vi "CreateInterface.vi"(6 "InterfaceName":string, 7 "Application":refnum<vi>, 8 "error in":errorcluster, 9 "Interface Folder":path, 10 "Parent Interfaces(ClassRef/Path)":variant[](array[variant]), 11 "New Interface Owner":refnum<vi>) -> (0 "error out":errorcluster, 1 "Interface":refnum<vi>, 2 "InterfaceName(Qualified Name)":string, 3 "InterfaceName(Non Qualified)":string, 4 "InterfacePath":path)   [LabVIEW 2020, in "InterfaceLibrary.lvlib"]
uses:
  <resource>/Framework/Providers/Open_GDS/ClassProviders/Common/InterfaceLibrary/InterfaceLibrary.lvlib
  <vilib>/numeric/Random Number (Range) U64.vi
  <vilib>/numeric/sub_Random U32.vi
  <resource>/Framework/Providers/_ClassSupport/Class Provider Support.lvlib
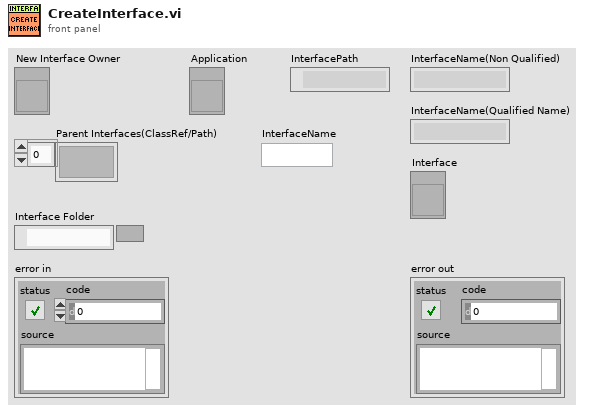
[diagram p1: front panel]
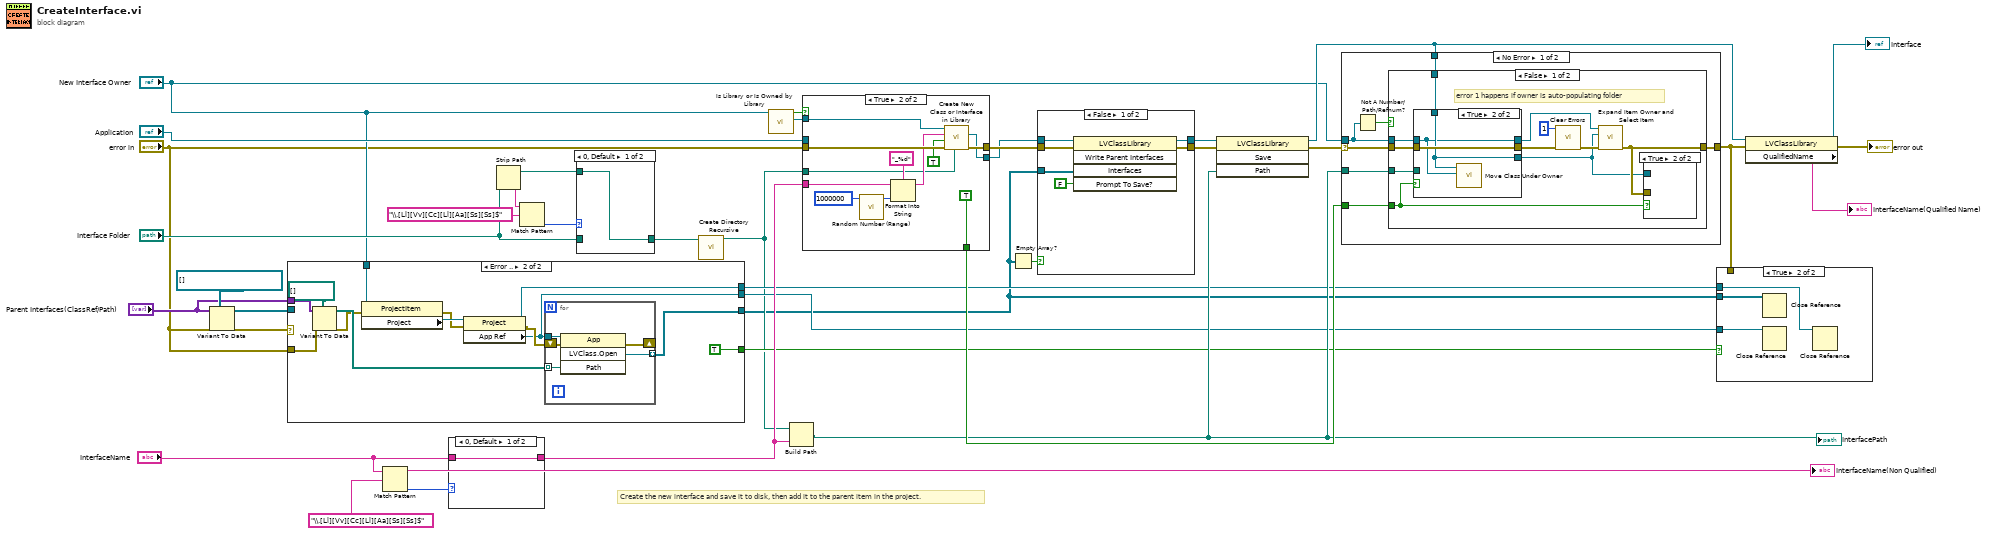
[diagram p0: block diagram]
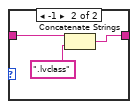
[diagram p4: hidden frame]
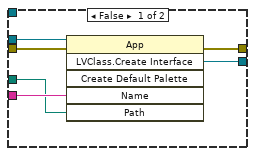
[diagram p6: hidden frame]
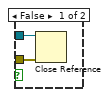
[diagram p7: hidden frame]
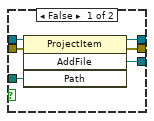
[diagram p8: hidden frame]
diagram:
  # "Create the new interface and save it to disk, then add it to the parent item in the project."
  n1 = Variant To Data(error in="error in", type=refnum<vi>[] [] ("Interface"), Variant="Parent Interfaces(ClassRef/Path)") -> (data=w11:refnum<vi>[], error out=w12:errorcluster)
  n2 = case shown="Error .." w12 {
    tunnel: [w39 w43] -> w1
    tunnel: w11 -> [w39 _]
    tunnel: "Parent Interfaces(ClassRef/Path)" -> [_ w51]
    tunnel: "New Interface Owner" -> [_ w50]
    tunnel: "error in" -> [_ w44]
    tunnel: [_ w42] -> w7
    tunnel: [_ w41] -> w6
    tunnel: [_ TRUE] -> w4
    frame No Error {
    }
    frame Error {
      n3 = Variant To Data(error in=w44, type=path[] [] ("Interface"), Variant=w51) -> (data=w48:path[], error out=w45:errorcluster)
      n4 = property class="ProjectItem"(reference=w50, error in=w45) -> (error out=w46:errorcluster, "Project"=w49:refnum<vi>)  [unwired: 1 out]
      n5 = property class="Project"(reference=w49, error in=w46) -> (reference out=w41:refnum<vi>, error out=w47:errorcluster, "App Ref"=w42:refnum<vi>)
      n6 = for {
        tunnel: w42 -> [w57]
        tunnel: w48 -> [w56] mode=indexing
        tunnel: [w54] -> w43 mode=indexing
        shift-right: [w53] -> _
        shift-left: w47 -> [w55]
        n7 = invoke class="App" method="LVClass.Open"(reference=w57, error in=w55, "Path"=w56) -> (error out=w53:errorcluster, "LVClass.Open"=w54:refnum<vi>)  [unwired: 1 in, 2 out]
      }
    }
  }
  n8 = Match Pattern(string="InterfaceName", regular expression="\\.[Ll][Vv][Cc][Ll][Aa][Ss][Ss]$") -> (before substring=→"InterfaceName(Non Qualified)":string, offset past match=w22:i32)  [unwired: 1 in, 2 out]
  n9 = case shown="0, Default" w22 {
    tunnel: "InterfaceName" -> [w58 w61]
    tunnel: [w58 w59] -> w20
    frame 0, Default {
    }
    frame -1 {
      n10 = Concatenate Strings(w61, ".lvclass" ("string")) -> (w59:string)
    }
  }
  n11 = Strip Path(path="Interface Folder") -> (stripped path=w24:path, name=w28:string)
  n12 = Match Pattern(string=w28, regular expression="\\.[Ll][Vv][Cc][Ll][Aa][Ss][Ss]$") -> (offset past match=w26:i32)  [unwired: 1 in, 3 out]
  n13 = case shown="0, Default" w26 {
    tunnel: "Interface Folder" -> [_ w63]
    tunnel: [w62 w63] -> w3
    tunnel: w24 -> [w62 _]
    frame 0, Default {
    }
    frame -1 {
    }
  }
  n14 = call <vilib>:"Create Directory Recursive.vi"("directory"=w3) -> ("directory copy"=w2:path)  [unwired: 4 in, 2 out]
  n15 = call <resource>:"Is Library or Is Owned by Library.vi"("ProjectItem"="New Interface Owner") -> ("Owning Library (or self)"=w33:refnum<vi>, "Is Library or Owned by Library?"=w32:bool)  [unwired: 9 in]
  n16 = Build Path(base path=w2, name or relative path=w20) -> (appended path=w14:path)
  "InterfacePath" <- w14
  n17 = case shown="True" w32 {
    tunnel: "error in" -> [w69 w81]
    tunnel: [w68 w80] -> w36
    tunnel: "Application" -> [w67 _]
    tunnel: w20 -> [w66 w75]
    tunnel: [w65 w78] -> w30
    tunnel: w33 -> [_ w79]
    tunnel: [_ TRUE] -> w29
    tunnel: w2 -> [w64 w70]
    frame False {
      n18 = invoke class="App" method="LVClass.Create Interface"(reference=w67, error in=w69, "Name"=w66, "Path"=w64) -> (error out=w68:errorcluster, "LVClass.Create Interface"=w65:refnum<vi>)  [unwired: 2 in, 4 out]
    }
    frame True {
      n19 = call-poly <vilib>:"Random Number (Range).vi"("upper bound (100)"=u64 1000000) -> ("number"=w72:u64)  [unwired: 10 in]
      n20 = Format Into String(format string="_%d", initial string=w75, w72) -> (resulting string=w74:string)  [unwired: 1 in, 1 out]
      n21 = call <vilib>:"Create New Class or Interface in Library.vi"("directory (empty)"=w70, "error in"=w81, "create interface"=TRUE, "new class file name"=w74, "library reference in"=w79) -> ("error out"=w80:errorcluster, "class reference"=w78:refnum<vi>)  [unwired: 4 in, 1 out]
    }
  }
  n22 = Empty Array?(array=w1) -> (empty?=w34:bool)
  n23 = case shown="False" w34 {
    tunnel: w36 -> [w87 w89]
    tunnel: [w86 w89] -> w37
    tunnel: w30 -> [w85 w88]
    tunnel: [w84 w88] -> w35
    tunnel: w1 -> [w82 _]
    frame False {
      n24 = invoke class="LVClassLibrary" method="Write Parent Interfaces"(reference=w85, error in=w87, "Interfaces"=w82, "Prompt To Save?"=FALSE) -> (reference out=w84:refnum<vi>, error out=w86:errorcluster)  [unwired: 1 in, 3 out]
    }
    frame True {
    }
  }
  n25 = invoke class="LVClassLibrary" method="Save"(reference=w35, error in=w37, "Path"=w14) -> (reference out=w17:refnum<vi>, error out=w38:errorcluster)  [unwired: 1 in, 2 out]
  n26 = case shown="No Error" w38 {
    selector: w38 -> [w96 w120]
    tunnel: "New Interface Owner" -> [w93 _]
    tunnel: w14 -> [w94 _]
    tunnel: [w95 w120] -> w5
    tunnel: w29 -> [w91 _]
    tunnel: w17 -> [w90 _]
    frame No Error {
      n27 = Not A Number/Path/Refnum?(number/path/refnum=w93) -> (NaN/Path/Refnum?=w92:bool)
      n28 = case shown="False" w92 {
        tunnel: w96 -> [w107 w119]
        tunnel: w94 -> [w102 _]
        tunnel: [w105 w119] -> w95
        tunnel: w93 -> [w99 _]
        tunnel: w91 -> [w97 _]
        tunnel: w90 -> [w98 _]
        frame False {
          # "error 1 happens if owner is auto-populating folder"
          n29 = case shown="True" w97 {
            tunnel: w107 -> [w115 w118]
            tunnel: [w114 w118] -> w106
            tunnel: [w113 w117] -> w103
            tunnel: w102 -> [w112 _]
            tunnel: [w111 w116] -> w101
            tunnel: w99 -> [w110 w116]
            tunnel: w98 -> [_ w117]
            frame False {
              n30 = invoke class="ProjectItem" method="AddFile"(reference=w110, error in=w115, "Path"=w112) -> (reference out=w111:refnum<vi>, error out=w114:errorcluster, "AddFile"=w113:refnum<vi>)  [unwired: 1 in, 1 out]
            }
            frame True {
              n31 = call <resource>:"Move Class Under Owner.vi"("Owner of New Class"=w116, "New Class"=w117) -> ()  [unwired: 9 in, 1 out]
            }
          }
          n32 = call <vilib>:"Clear Errors.vi"("error in (no error)"=w106, "specific error code to clear (0: all)"=1) -> ("error out"=w104:errorcluster)  [unwired: 4 in, 1 out]
          n33 = call <resource>:"Expand Item Owner and Select Item.vi"("error in"=w104, "New Item"=w103, "New Item Owner"=w101) -> ("error out"=w105:errorcluster)  [unwired: 8 in]
          n34 = case shown="True" w97 {
            tunnel: w105 -> [w109 _]
            tunnel: w103 -> [w108 _]
            frame False {
              n35 = Close Reference(reference=w108, error in (no error)=w109) -> ()  [unwired: 1 out]
            }
            frame True {
            }
          }
        }
        frame True {
        }
      }
    }
    frame Error {
    }
  }
  n36 = case shown="True" w4 {
    tunnel: w7 -> [_ w123]
    tunnel: w6 -> [_ w122]
    tunnel: w5 -> [_ _]
    tunnel: w1 -> [_ w121]
    frame False {
    }
    frame True {
      n37 = Close Reference(reference=w121) -> ()  [unwired: 1 in, 1 out]
      n38 = Close Reference(reference=w123) -> ()  [unwired: 1 in, 1 out]
      n39 = Close Reference(reference=w122) -> ()  [unwired: 1 in, 1 out]
    }
  }
  n40 = property class="LVClassLibrary"(reference=w17, error in=w5) -> (reference out=→"Interface":refnum<vi>, error out=→"error out":errorcluster, "QualifiedName"=→"InterfaceName(Qualified Name)":string)
